vi "Poly_Timer.vi"   [LabVIEW 2012]
doc: "Timer function, made unique by specified \"Timer\" value."
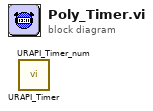
[diagram p0: block diagram]
diagram:
  n1 = call <userlib>:"URAPI_Timer.vi"() -> ()  [unwired: 4 in, 2 out]
  n2 = call <userlib>:"URAPI_Timer_num.vi"() -> ()  [unwired: 4 in, 2 out]
